vi "s-lab第9章 图形显示1-9.vi"() -> ()   [LabVIEW 2013]
uses:
  <vilib>/express/express analysis/Spectral/Block/exnSpectralBlock spectral measurements RMS poly.vi
  <vilib>/express/express analysis/Spectral/Block/exnSpectralBlock spectral measurements RMS DDT.vi
  <vilib>/express/express analysis/Spectral/XNode/ExpressSpectralMeasurementsBlockNode.xnode
  <vilib>/measure/NI_MABase.lvlib
  <vilib>/measure/NI_MAPro.lvlib
  <vilib>/Analysis/NI_AALBase.lvlib
panel:
  out "XY图":T1(graph)
  out "波形图表 9":dynamicdata(graph)
  in  "停止 7":bool
  in  "停止 6":bool
  in  "频率38":dbl
  in  "幅值":dbl
  out "滤波后的波形图":dynamicdata(graph)
  out "波形图表 8":waveform(dbl)(graph)
  out "波形图表 7":waveform(dbl)(graph)
  in  "停止 5":bool
  in  "幅值":dbl
  in  "频率":dbl
  in  "停止 4":bool
  out "波形图表 6":waveform(dbl)(graph)
  in  "相位":dbl
  in  "幅值":dbl
  in  "频率":dbl
  in  "信号类型":u16(ring) items=["正弦波", "三角波", "方波", "锯齿波"]
  out "波形图表 5":dynamicdata(graph)
  in  "停止 3":bool
  in  "噪声幅值":dbl
  in  "频率":dbl
  in  "幅值":dbl
  out "波形图表 4":dynamicdata(graph)
  out "幅值":dbl
  out "频率":dbl
  in  "停止 2":bool
  in  "幅值调节":dbl(knob) scale=0.0..10.0
  in  "频率调节":dbl(knob) scale=0.0..10.0
  out "波形图表 3":waveform(dbl)(graph)
  out "波形图表 2":dbl(graph)
  in  "停止":bool
  out "波形图表":dbl(graph)
  # "例 1"
  # "例 2"
  # "例 3"
  # "例 4"
  # "例 5"
  # "数字示波器"
  # "例 6"
  # "例 7"
  # "例 8"
  # "例 9"
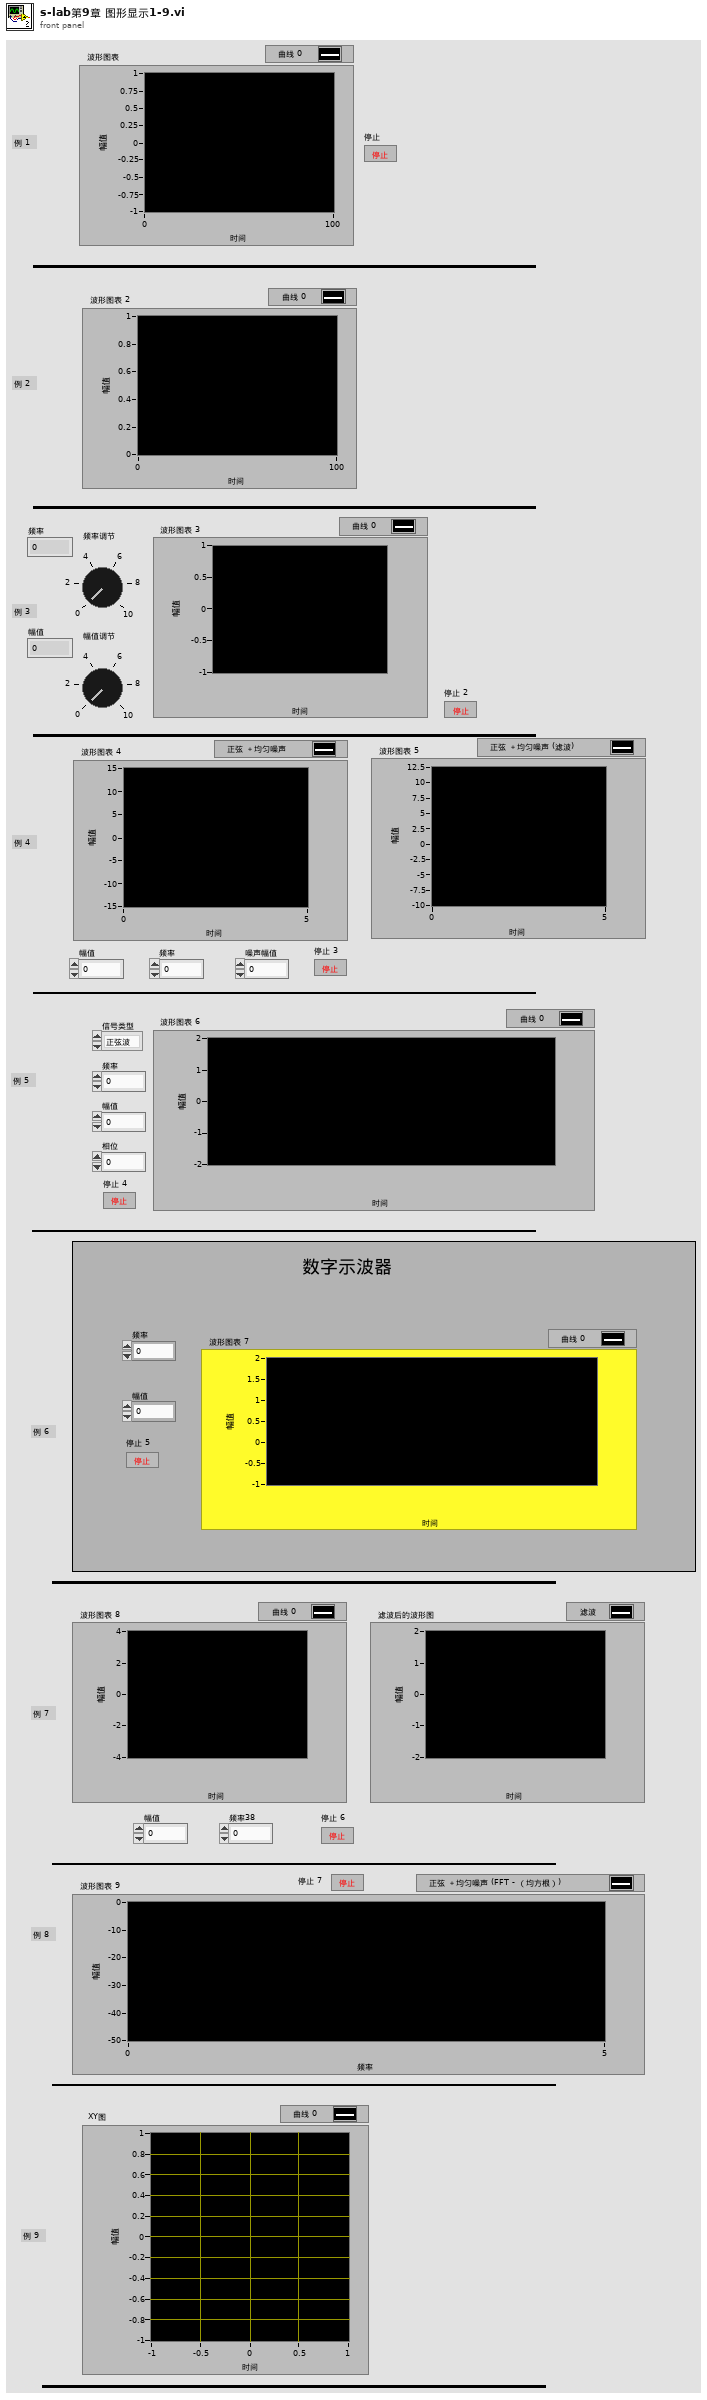
[diagram p1: front panel]
types:
  T1 = cluster{"Sinusoidal Pattern":dbl[], "Sinusoidal Pattern":dbl[]}
  T2 = cluster{"averaging mode":u16, "weighting mode":u16, "number of averages":u32}
  T3 = cluster{"dB On (F)":bool, "unwrap phase (F)":bool, "convert to degree (F)":bool}
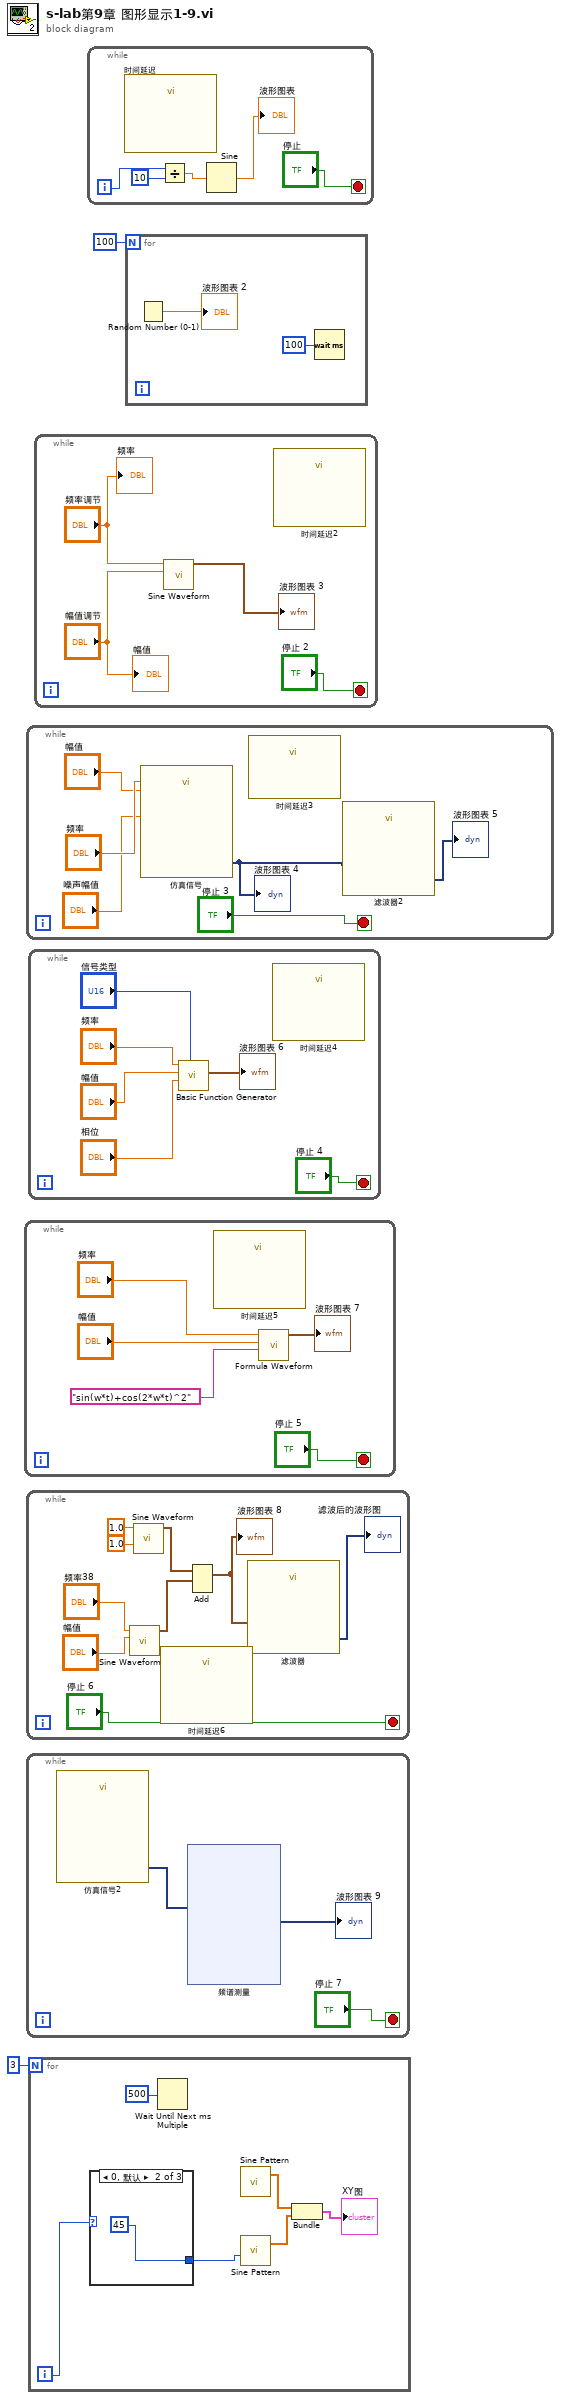
[diagram p0: block diagram]
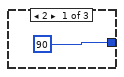
[diagram p2: hidden frame]
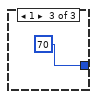
[diagram p3: hidden frame]
diagram:
  n1 = while {
    stop <- "停止 5" stop-if-true
    n2 = call "时间延迟5"() -> ()  [unwired: 11 in, 1 out]
    n3 = call <vilib>:"Formula Waveform.vi"("formula"="sin(w*t)+cos(2*w*t)^2", "amplitude"="幅值", "frequency"="频率") -> ("signal out"=→"波形图表 7":waveform(dbl))  [unwired: 7 in, 1 out]
  }
  n4 = while {
    stop <- "停止 3" stop-if-true
    n5 = call "仿真信号"("Frequency"="频率", "Amplitude"="幅值", "噪声幅值"="噪声幅值") -> ("正弦与均匀噪声"=w9:dynamicdata)  [unwired: 11 in, 1 out]
    "波形图表 4" <- w9
    n6 = call "时间延迟3"() -> ()  [unwired: 11 in, 1 out]
    n7 = call "滤波器2"("Signal"=w9) -> ("Filtered Signal"=→"波形图表 5":dynamicdata)  [unwired: 9 in, 1 out]
  }
  n8 = while {
    stop <- "停止 6" stop-if-true
    n9 = call <vilib>:"Sine Waveform.vi"("amplitude"="幅值", "frequency"="频率38") -> ("signal out"=w16:waveform(dbl))  [unwired: 8 in, 1 out]
    n10 = call <vilib>:"Sine Waveform.vi"("amplitude"=1.0, "frequency"=1.0) -> ("signal out"=w17:waveform(dbl))  [unwired: 8 in, 1 out]
    n11 = call "时间延迟6"() -> ()  [unwired: 11 in, 1 out]
    n12 = Add(1:w16, 2:w17) -> (0:w15:waveform(dbl))  [unwired: 1 in, 1 out]
    "波形图表 8" <- w15
    n13 = call "滤波器"("Signal"=w15) -> ("Filtered Signal"=→"滤波后的波形图":dynamicdata)  [unwired: 9 in, 1 out]
  }
  n14 = while {
    stop <- "停止 7" stop-if-true
    n15 = call "仿真信号2"() -> ("正弦与均匀噪声"=w25:dynamicdata)  [unwired: 14 in, 1 out]
    n16 = xnode "频谱测量"("信号"=w25) -> ("FFT - （均方根）"=→"波形图表 9":dynamicdata)  [unwired: 2 in, 3 out]
  }
  n17 = while {
    stop <- "停止 4" stop-if-true
    n18 = call <vilib>:"Basic Function Generator.vi"("signal type"="信号类型", "phase"="相位", "amplitude"="幅值", "frequency"="频率") -> ("signal out"=→"波形图表 6":waveform(dbl))  [unwired: 5 in, 2 out]
    n19 = call "时间延迟4"() -> ()  [unwired: 11 in, 1 out]
  }
  n20 = for {
    N: 3 -> [_]
    i -> [w48]
    n21 = case shown="0, 默认" w48 {
      tunnel: [90 45 70] -> w43
      frame 2 {
      }
      frame 0, Default {
      }
      frame 1 {
      }
    }
    n22 = Wait Until Next ms Multiple(millisecond multiple=u32 500 ("毫秒倍数")) -> ()  [unwired: 1 out]
    n23 = call <vilib>:"Sine Pattern.vi"() -> ("Sinusoidal Pattern"=w47:dbl[])  [unwired: 4 in, 1 out]
    n24 = call <vilib>:"Sine Pattern.vi"("phase(degrees)"=w43) -> ("Sinusoidal Pattern"=w46:dbl[])  [unwired: 3 in, 1 out]
    n25 = Bundle("Sinusoidal Pattern"=w47, "Sinusoidal Pattern"=w46) -> (→"XY图":T1)  [unwired: 1 in]
  }
  n26 = while {
    stop <- "停止 2" stop-if-true
    n27 = call <vilib>:"Sine Waveform.vi"("amplitude"="幅值调节", "frequency"="频率调节") -> ("signal out"=→"波形图表 3":waveform(dbl))  [unwired: 8 in, 1 out]
    n28 = call "时间延迟2"() -> ()  [unwired: 11 in, 1 out]
    "幅值" <- "幅值调节"
    "频率" <- "频率调节"
  }
  n29 = while {
    i -> [w59]
    stop <- "停止" stop-if-true
    n30 = call "时间延迟"() -> ()  [unwired: 11 in, 1 out]
    n31 = Divide(x=w59, y=10) -> (x/y=w57:dbl)
    n32 = Sine(x=w57) -> (sin(x)=→"波形图表":dbl)
  }
  n33 = for {
    N: 100 -> [_]
    n34 = Random Number (0-1)() -> (number: 0 to 1=→"波形图表 2":dbl)
    n35 = Wait (ms)(milliseconds to wait=u32 100 ("等待时间（毫秒）")) -> ()  [unwired: 1 out]
  }
